vi "Init_Test.vi"(8 "error in (no error)":errorcluster caption="entrée d'erreur (pas d'erreur)", 11 "Test (Default) en entrée":refnum<class "Test (Default).lvclass">) -> (0 "error out":errorcluster caption="sortie d'erreur", 3 "Test (Default) en sortie":refnum<class "Test (Default).lvclass">)   [LabVIEW 2020, in "Library Test.lvlib" / "Test (Default).lvclass"]
uses:
  Test (Default).lvclass
  Test (Default).lvclass/Test (Default).ctl
  Core/Actors/Actor_Log/Actor_Log/Actor_Log Messages/Log Msg/Log Msg.lvclass/Log Msg.ctl
  <vilib>/ActorFramework/Message Enqueuer/Message Enqueuer.lvclass/Message Enqueuer.ctl
  <vilib>/ActorFramework/Message Enqueuer/Enqueue.vi
  Core/Actors/Actor_Log/Actor_Log/Actor_Log Messages/Log Msg/Log Msg.lvclass
  C:/Program Files (x86)/National Instruments/LabVIEW 2020/vi.lib/ActorFramework/Message/Message.lvclass
  <vilib>/ActorFramework/Message Priority Queue/Priority Enqueue.vi
  Commun VI/Library Commun.lvlib
  Instrument/Instrument (Default)/Class Instrument (Default).lvclass
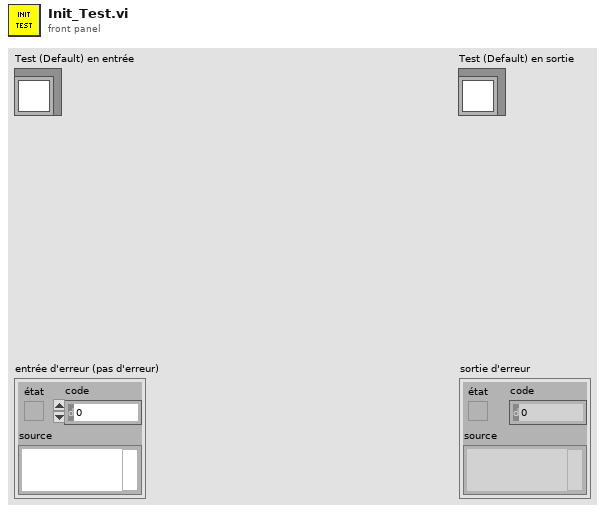
[diagram p1: front panel]
types:
  T1 = enum16{"Init", "Add Actor", "Delete Actor", "Get Actor Queue", "Get Log Actor Queue", "List all actors"}
  T2 = enum16{"Get Test Class", "Set Test object", "Get Test object", "List Test", "Init"}
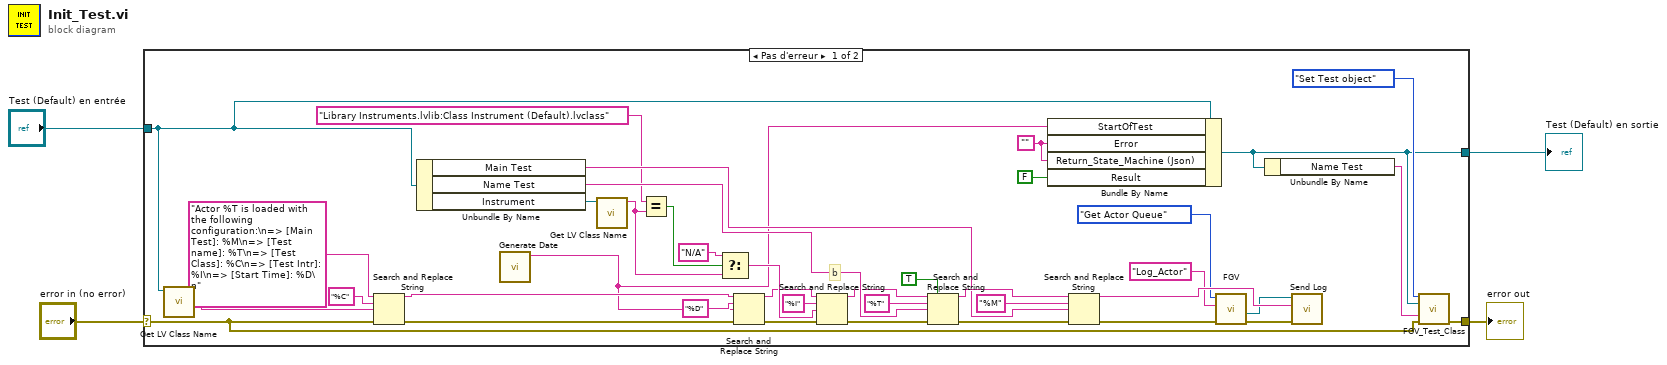
[diagram p0: block diagram]
diagram:
  n1 = case shown="Pas d'erreur" "error in (no error)" {
    selector: "error in (no error)" -> [w6 w45]
    tunnel: [w39 w45] -> w2
    tunnel: [w38 w44] -> w3
    tunnel: "Test (Default) en entrée" -> [w18 w44]
    frame No Error {
      w43 = "" ("Data Test.Error")
      # "b"
      n2 = call <vilib>:"Get LV Class Name.vi"("object"=w18) -> ("class name"=w17:string)  [unwired: 9 in, 1 out]
      n3 = Search and Replace String(input string="Actor %T is loaded with the following configuration:\n=> [Main Test]: %M\n=> [Test name]: %T\n=> [Test Class]: %C\n=> [Test Intr]: %I\n=> [Start Time]: %D\n", search string="%C", replace string=w17, error in=w6) -> (result string=w9:string, error out=w11:errorcluster)  [unwired: 4 in, 2 out]
      n4 = Unbundle By Name(w18) -> ("Main Test"=w35:string, "Name Test"=w33:string, "Instrument"=w30:refnum<class "Class Instrument (Default).lvclass">)
      n5 = call "Generate Date.vi"() -> ("chaîne de date/heure"=w5:string)  [unwired: 11 in]
      n6 = call <vilib>:"Get LV Class Name.vi"("object"=w30) -> ("class name"=w20:string)  [unwired: 9 in, 1 out]
      n7 = Equal?(x="Library Instruments.lvlib:Class Instrument (Default).lvclass" ("y"), y=w20) -> (x = y?=w22:bool)
      n8 = Select(t="N/A", s=w22, f=w20) -> (s? t:f=w19:string)
      n9 = Search and Replace String(input string=w9, search string="%D", replace string=w5, error in=w11) -> (result string=w8:string, error out=w10:errorcluster)  [unwired: 4 in, 2 out]
      n10 = Search and Replace String(input string=w8, search string="%I", replace string=w19, error in=w10) -> (result string=w32:string, error out=w31:errorcluster)  [unwired: 4 in, 2 out]
      n11 = Search and Replace String(replace all?=TRUE ("replace all? (F)"), input string=w32, search string="%T", replace string=w33, error in=w31) -> (result string=w36:string, error out=w34:errorcluster)  [unwired: 3 in, 2 out]
      n12 = Bundle By Name(cluster=w18, "StartOfTest"=w5, "Error"=w43, "Return_State_Machine (Json)"=w43, "Result"=FALSE ("Data Test.Result")) -> (w38:refnum<class "Test (Default).lvclass">)
      n13 = Search and Replace String(input string=w36, search string="%M", replace string=w35, error in=w34) -> (result string=w37:string, error out=w13:errorcluster)  [unwired: 4 in, 2 out]
      n14 = call "FGV.vi"("error in (no error)"=w13, "Actor name"="Log_Actor", "Action"=T1."Get Actor Queue") -> ("error out"=w12:errorcluster, "Actor's Queue Out"=w14:refnum<class "Message Enqueuer.lvclass">)  [unwired: 6 in, 1 out]
      n15 = Unbundle By Name(w38) -> ("Name Test"=w40:string)
      n16 = call "Send Log.vi"("error in (no error)"=w12, "String to add"=w37, "Message Enqueuer"=w14) -> ()  [unwired: 7 in, 2 out]
      n17 = call "FGV_Test_Class.vi"("Action"=T2."Set Test object", "Test"=w38, "Test Name"=w40, "error in (no error)"=w6) -> ("error out"=w39:errorcluster)  [unwired: 8 in, 3 out]
    }
    frame Error {
    }
  }
  "error out" <- w2
  "Test (Default) en sortie" <- w3
